vi "Fetch Analog Waveform.vi"(8 "error in (no error)":errorcluster, 9 "Timeout (10000 ms)":u32=10000, 10 "Source (0: Channel 1)":u16(ring) items=["Channel 1", "Channel 2", "Channel 3", "Channel 4", "Math"], 11 "VISA resource name":refnum<visa-resource-name>) -> (0 "error out":errorcluster, 2 "Waveform Data":waveform(dbl)(graph), 3 "VISA resource name out":refnum<visa-resource-name>)   [LabVIEW 2021, in "Agilent 6000 Series.lvlib"]
doc: "Returns the waveform the oscilloscope acquired for the specified channel. The waveform is from an acquisition that you initiate prior to calling this VI.\n\nYou use the Initiate VI to start an acquisition on the channels that you enable with the <B>Configure Channel</B> VI. The oscilloscope acquires waveforms for the enabled channels concurrently. You must call this VI separately for each enabled channel to obtain the waveforms.\n\nYou can call the <B>ag6000a Read Waveforms</B> VI instead of using low level VIs.\n\n<B>Note</B> This VI does not check the instrument status. Typically, you call this VI only in a sequence of calls to other low-level instrument driver VIs. The sequence performs one operation. You use the low-level VIs to optimize one or more aspects of interaction with the instrument."
uses:
  Agilent 6000 Series.lvlib
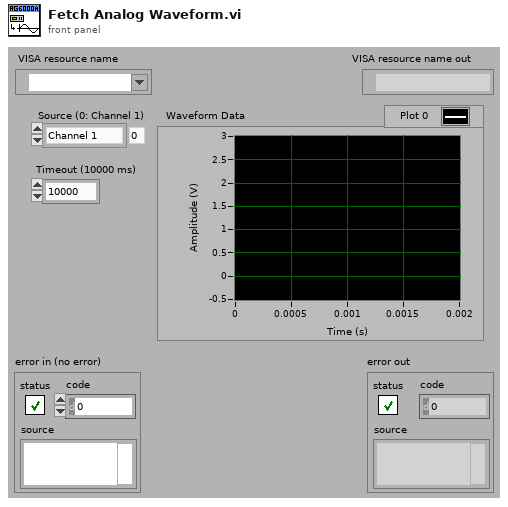
[diagram p1: front panel]
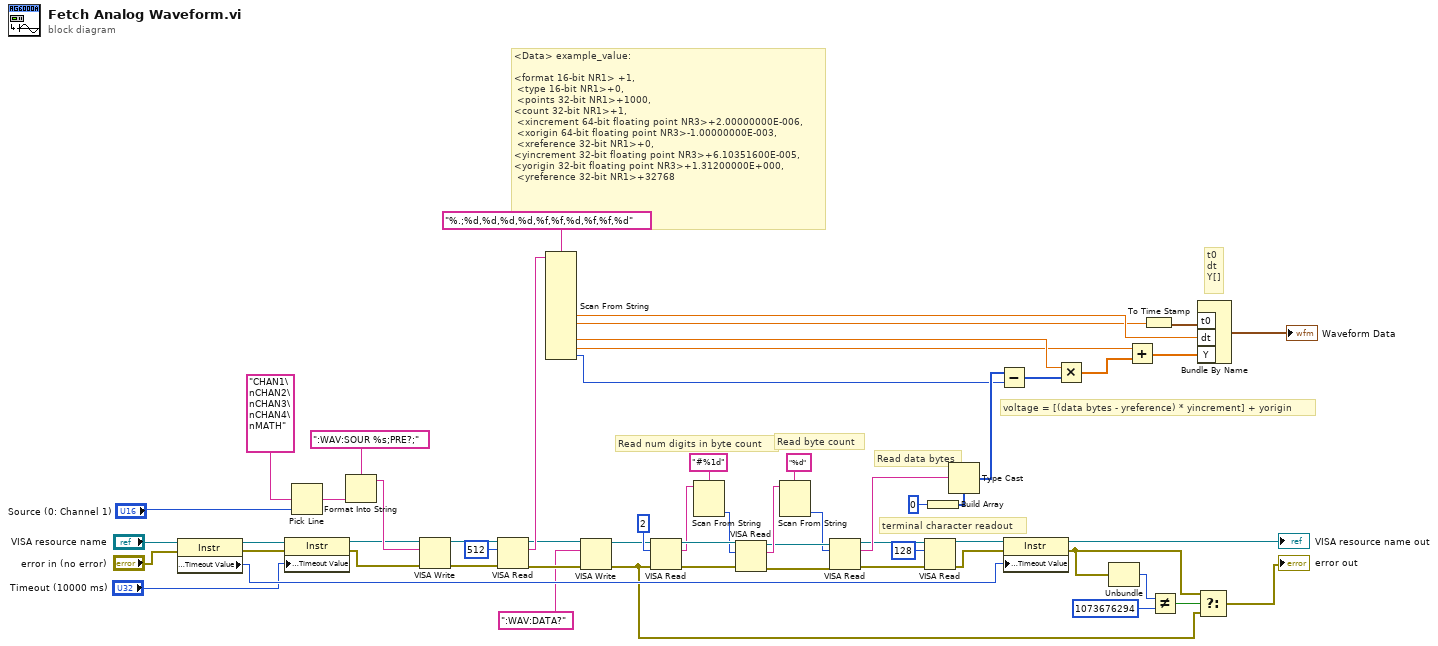
[diagram p0: block diagram]
diagram:
  # "voltage = [(data bytes - yreference) * yincrement] + yorigin"
  # "t0\ndt\nY[]"
  # "<Data> example_value:\n\n<format 16-bit NR1> +1,\n <type 16-bit NR1>+0,\n <points 32-bit NR1>+1000, \n<count 32-bit NR1>+1,\n <xincrement 64-bit floating point NR3>+2.00000000E-006,\n <xorigin 64-bit floating point NR3>-1.00000000E-003,\n <xreference 32-bit NR1>+0, \n<yincrement 32-bit floating point NR3>+6.10351600E-005, \n<yorigin 32-bit floating point NR3>+1.31200000E+000,\n <yreference 32-bit NR1>+32768"
  # "terminal character readout"
  # "Read data bytes"
  # "Read num digits in byte count"
  # "Read byte count"
  n1 = property on="Property Node" class="Instr"(reference="VISA resource name", error in="error in (no error)") -> (reference out=w44:refnum<visa-resource-name>, error out=w43:errorcluster, "General Settings:Timeout Value"=w45:u32)
  n2 = property on="Property Node" class="Instr"(reference=w44, error in=w43, "General Settings:Timeout Value"="Timeout (10000 ms)") -> (reference out=w41:refnum<visa-resource-name>, error out=w40:errorcluster)
  n3 = Pick Line(multi-line string="CHAN1\nCHAN2\nCHAN3\nCHAN4\nMATH", line index="Source (0: Channel 1)") -> (output string=w53:string)  [unwired: 1 in]
  n4 = Format Into String(format string=":WAV:SOUR %s;PRE?;", w53) -> (resulting string=w52:string)  [unwired: 2 in, 1 out]
  n5 = VISA Write(VISA resource name=w41, write buffer=w52, error in (no error)=w40) -> (VISA resource name out=w50:refnum<visa-resource-name>, error out=w51:errorcluster)  [unwired: 1 out]
  n6 = VISA Read(VISA resource name=w50, byte count=u32 512, error in (no error)=w51) -> (VISA resource name out=w39:refnum<visa-resource-name>, read buffer=w48:string, error out=w38:errorcluster)  [unwired: 1 out]
  n7 = Scan From String(format string="%.;%d,%d,%d,%d,%f,%f,%d,%f,%f,%d", input string=w48) -> (output 5=w9:dbl, output 6=w8:dbl, output 8=w3:dbl, output 9=w1:dbl, output 10=w5:i32)  [unwired: 17 in, 3 out]
  n8 = VISA Write(VISA resource name=w39, write buffer=":WAV:DATA?", error in (no error)=w38) -> (VISA resource name out=w30:refnum<visa-resource-name>, error out=w12:errorcluster)  [unwired: 1 out]
  n9 = VISA Read(VISA resource name=w30, byte count=u32 2, error in (no error)=w12) -> (VISA resource name out=w33:refnum<visa-resource-name>, read buffer=w31:string, error out=w34:errorcluster)  [unwired: 1 out]
  n10 = Scan From String(format string="#%1d", input string=w31) -> (output 1=w32:i32)  [unwired: 3 in, 3 out]
  n11 = VISA Read(VISA resource name=w33, byte count=w32, error in (no error)=w34) -> (VISA resource name out=w26:refnum<visa-resource-name>, read buffer=w28:string, error out=w27:errorcluster)  [unwired: 1 out]
  n12 = Scan From String(format string="%d", input string=w28) -> (output 1=w24:i32)  [unwired: 3 in, 3 out]
  n13 = VISA Read(VISA resource name=w26, byte count=w24, error in (no error)=w27) -> (VISA resource name out=w22:refnum<visa-resource-name>, read buffer=w25:string, error out=w23:errorcluster)  [unwired: 1 out]
  n14 = VISA Read(VISA resource name=w22, byte count=u32 128, error in (no error)=w23) -> (VISA resource name out=w21:refnum<visa-resource-name>, error out=w20:errorcluster)  [unwired: 2 out]
  n15 = Build Array(u16 0) -> (w59:u16[])
  n16 = Type Cast(type=w59, x=w25) -> (*(type *) &x=w6:u16[])
  n17 = Subtract(x=w6, y=w5) -> (x-y=w4:i32[])
  n18 = property on="Property Node" class="Instr"(reference=w21, error in=w20, "General Settings:Timeout Value"=w45) -> (reference out=→"VISA resource name out":refnum<visa-resource-name>, error out=w15:errorcluster)
  n19 = Multiply(x=w3, y=w4) -> (x*y=w2:dbl[])
  n20 = Unbundle(w15) -> ("code"=w18:i32)  [unwired: 2 out]
  n21 = Add(x=w1, y=w2) -> (x+y=w7:dbl[])
  n22 = To Time Stamp(1:w8) -> (0:w11:timestamp)
  n23 = Not Equal?(x=w18, y=1073676294) -> (x != y?=w16:bool)
  n24 = Bundle By Name ("Build Waveform")("t0"=w11, "dt"=w9, "Y"=w7) -> (→"Waveform Data":waveform(dbl))  [unwired: 1 in]
  n25 = Select(t=w15, s=w16, f=w12) -> (s? t:f=→"error out":errorcluster)
